vi "CRYRunning Jump Logic.vi"(0 "Step Configure":T1={"No.VI"=0, "Category"="", "StepName"="", "Seq setup flattened"="", "Comment"="", "Steps config."=[], "Jump config"=[], "Start"=0.0, "Increment"=0.0, "Name"="Pa", "Unit"="Pa", "Y data"=1, "Y prefix"="", "Y dB ref"=1.0, "Y unit"="", "Repeat State Array"=[]} {"Repeat State Array"."Start" format="%#_5g"; "Y dB ref" format="%.1f"; "Y data" items=["dB", "Lin"]; "Start" format="%#_5g"}, 1 "Pass?":bool, 11 "Step pointer in":i32, 12 "Step execution count":i32, 13 "Allowed-to-run steps mask":bool[](array[boolean])) -> (4 "Step pointer out":i32, 15 "execution count out":i32)   [LabVIEW 2013]
uses:
  Typedef Control/CRYStep.ctl
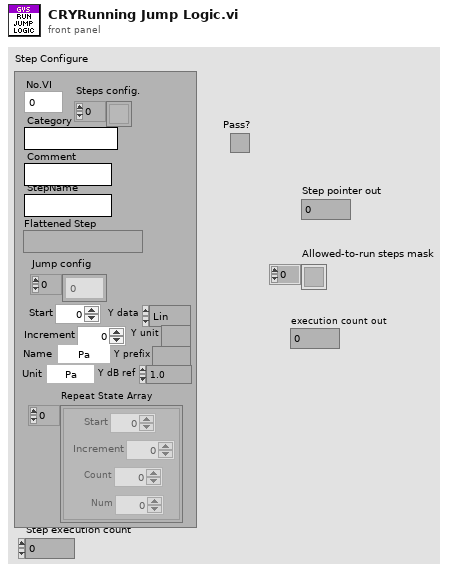
[diagram p1: front panel]
types:
  T1 = typedef "CRYStep.ctl" = cluster{"No.VI":i32, "Category":string, "StepName":string, "Seq setup flattened":string, "Comment":string, "Steps config.":bool[], "Jump config":i32[], "Start":dbl, "Increment":dbl, "Name":string, "Unit":string, "Y data":u16, "Y prefix":string, "Y dB ref":dbl, "Y unit":string, "Repeat State Array":cluster{"Start":dbl, "Increment":dbl, "Count":i32, "Num":i32}[]}
  T2 = typedef "CRYData Cluster Array.ctl" = T3[]
  T3 = typedef "CRYData Cluster.ctl" = cluster{"Name":string, "Curve":cluster{"x":dbl, "y":dbl, "z":dbl}[], "X data":u16, "Y data":u16, "Z data":u16, "X axis":u16, "Y axis":u16, "Z axis":u16, "X unit":string, "Y unit":string, "Z unit":string, "X dB ref":dbl, "Y dB ref":dbl, "Z dB ref":dbl, "single val":bool, "protected":bool, "display X":bool, "display Y":bool, "display Z":bool, "Test Info":string, "Step No.":i32, "Plot Settings":cluster{"Color":u32, "Interpolation":u8, "Point Style":u8, "Line Style":u8, "Point Color":u32, "Line Width":u8, "Bar Plot Style":u8, "Fill To":i16}, "AutoProtect":bool}
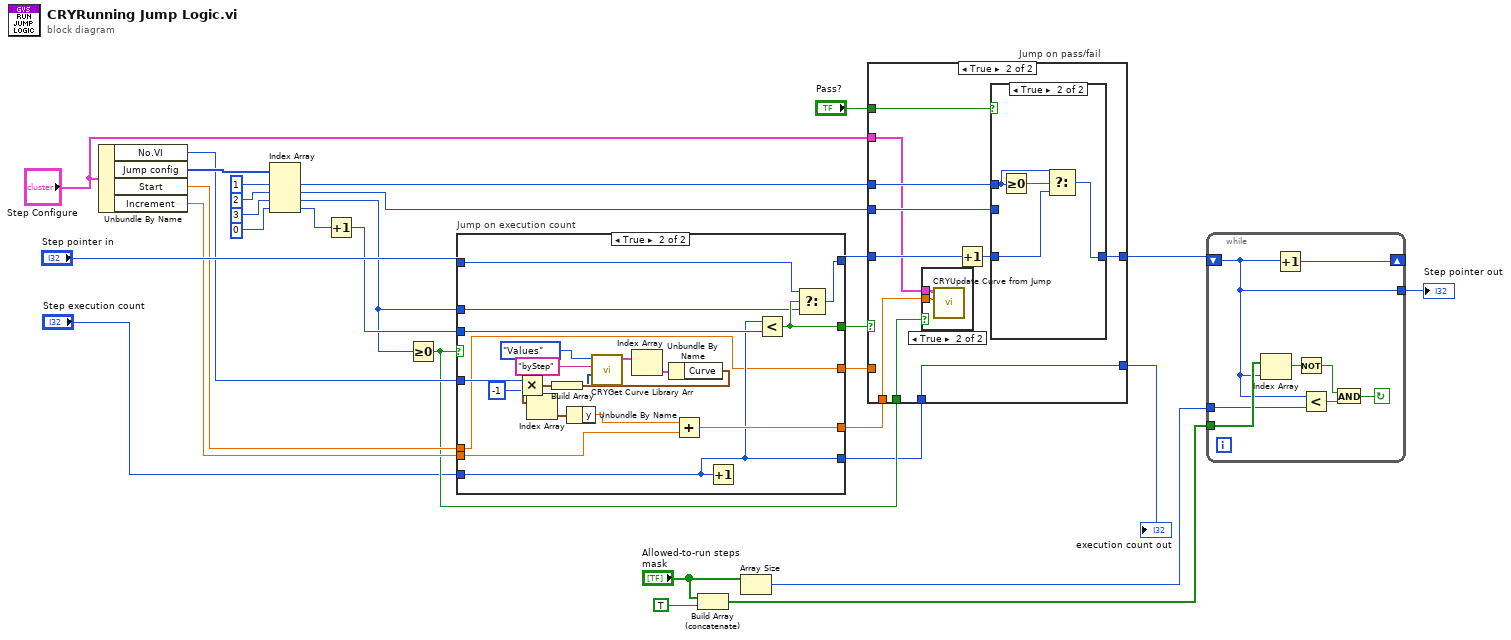
[diagram p0: block diagram]
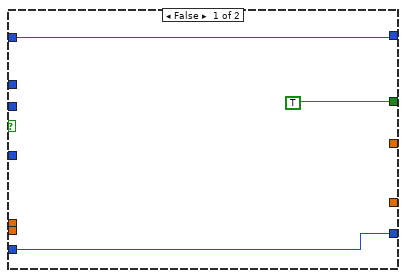
[diagram p2: hidden frame]
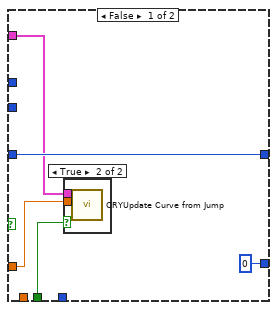
[diagram p3: hidden frame]
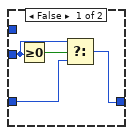
[diagram p6: hidden frame]
diagram:
  n1 = Unbundle By Name("Step Configure") -> ("No.VI"=w10:i32, "Jump config"=w15:i32[], "Start"=w9:dbl, "Increment"=w8:dbl)
  n2 = Index Array(array=w15, index #1=1 ("index"), index #2=2 ("index"), index #3=3 ("index"), index #4=0 ("index")) -> (element #1=w14:i32, element #2=w13:i32, element #3=w12:i32, element #4=w11:i32)
  n3 = Increment(x=w11) -> (x+1=w20:i32)
  n4 = Greater Or Equal To 0?(x=w12) -> (x >= 0?=w5:bool)
  n5 = case "Jump on execution count" shown="True" w5 {
    tunnel: w20 -> [_ w53]
    tunnel: w12 -> [_ w49]
    tunnel: "Step pointer in" -> [w33 w50]
    tunnel: [w33 w52] -> w29
    tunnel: [TRUE w51] -> w28
    tunnel: w10 -> [_ w39]
    tunnel: w9 -> [_ w34]
    tunnel: w8 -> [_ w37]
    tunnel: [_ w36] -> w6
    tunnel: "Step execution count" -> [w31 w35]
    tunnel: [w31 w35] -> w3
    tunnel: [_ w34] -> w1
    frame False {
    }
    frame True {
      n6 = Multiply(x=w39, y=-1) -> (x*y=w41:i32)
      n7 = Build Array(w41) -> (w44:i32[])
      n8 = call "CRYGet Curve Library Arr.vi"("Index"=w44, "sOption"="byStep", "Type In"=enum16{"Curves", "Values", "Results", "WFM"}."Values") -> ("Curves/Values"=w45:T2)  [unwired: 6 in, 2 out]
      n9 = Index Array(array=w45) -> (element=w46:T3)  [unwired: 1 in]
      n10 = Unbundle By Name(w46) -> ("Curve"=w47:cluster{"x":dbl, "y":dbl, "z":dbl}[])
      n11 = Index Array(array=w47) -> (element=w48:cluster{"x":dbl, "y":dbl, "z":dbl})  [unwired: 1 in]
      n12 = Unbundle By Name(w48) -> ("y"=w38:dbl)
      n13 = Add(x=w38, y=w37) -> (x+y=w36:dbl)
      n14 = Increment(x=w35) -> ()  [unwired: 1 out]
      n15 = Less?(x=w35, y=w53) -> (x < y?=w51:bool)
      n16 = Select(t=w50, s=w51, f=w49) -> (s? t:f=w52:i32)
    }
  }
  n17 = Build Array (concatenate)("Allowed-to-run steps mask", TRUE) -> (w25:bool[])
  n18 = Array Size(array="Allowed-to-run steps mask") -> (size(s)=w22:i32)
  n19 = case "Jump on pass/fail" shown="True" w28 {
    tunnel: w29 -> [w58 w65]
    tunnel: [w58 w67] -> w24
    tunnel: "Pass?" -> [_ w70]
    tunnel: w13 -> [_ w69]
    tunnel: w14 -> [_ w68]
    tunnel: "Step Configure" -> [w56 w64]
    tunnel: w6 -> [_ w63]
    tunnel: w5 -> [w55 w62]
    tunnel: w3 -> [_ w61]
    tunnel: [0 ("Step execution count") w61] -> w2
    tunnel: w1 -> [w54 _]
    frame False {
      n20 = case shown="True" w55 {
        tunnel: w56 -> [_ w60]
        tunnel: w54 -> [_ w59]
        frame False {
        }
        frame True {
          n21 = call "CRYUpdate Curve from Jump.vi"("Y Value"=w59, "Step Configure"=w60) -> ()  [unwired: 9 in, 1 out]
        }
      }
    }
    frame True {
      n22 = case shown="True" w62 {
        tunnel: w64 -> [_ w72]
        tunnel: w63 -> [_ w71]
        frame False {
        }
        frame True {
          n23 = call "CRYUpdate Curve from Jump.vi"("Y Value"=w71, "Step Configure"=w72) -> ()  [unwired: 9 in, 1 out]
        }
      }
      n24 = Increment(x=w65) -> (x+1=w66:i32)
      n25 = case shown="True" w70 {
        tunnel: w69 -> [w73 _]
        tunnel: w68 -> [_ w77]
        tunnel: w66 -> [w75 w79]
        tunnel: [w74 w78] -> w67
        frame False {
          n26 = Greater Or Equal To 0?(x=w73) -> (x >= 0?=w76:bool)
          n27 = Select(t=w73, s=w76, f=w75) -> (s? t:f=w74:i32)
        }
        frame True {
          n28 = Greater Or Equal To 0?(x=w77) -> (x >= 0?=w80:bool)
          n29 = Select(t=w77, s=w80, f=w79) -> (s? t:f=w78:i32)
        }
      }
    }
  }
  "execution count out" <- w2
  n30 = while {
    tunnel: [w81] -> w21
    tunnel: w22 -> [w86]
    shift-left: w24 -> [w81]
    shift-right: [w87] -> _
    tunnel: w25 -> [w88]
    stop <- w84 continue-if-true
    n31 = Index Array(array=w88, index=w81) -> (element=w83:bool)
    n32 = Increment(x=w81) -> (x+1=w87:i32)
    n33 = Not(x=w83) -> (.not. x?=w82:bool)
    n34 = Less?(x=w81, y=w86) -> (x < y?=w85:bool)
    n35 = And(x=w82, y=w85) -> (x .and. y?=w84:bool)
  }
  "Step pointer out" <- w21
